vi "WSS.Generate.Digital.vi"(8 "Man Ctrl Bit 1":bool, 9 "Man Ctrl Bit 0":bool, 10 "Manual Control":bool, 11 "LF Wheel Speed Sensor Settings":T1={"ACTIVE EDGE"=TRUE, "ACTIVE TICKS"=0, "INACTIVE TICKS"=0, "Data"=0, "Sensor Type"=0}) -> (1 "Bit1":bool, 2 "Bit0":bool)   [LabVIEW 2015, in "Speciality FPGA IO.lvlib"]
doc: "This VI Simulates Wheel Speed Sensors for Unidirectional, Bidirectional - Bosch, and Bidirectional Conti. Sensor Type is:\n0 - Unidirectional\n1 - Bidirectional Bosch\n2 - Bidirectional Continental. The output of the VI is two digital bits that correspond to the following current levels when paired with an OW-902 module:\nBit 0 Bit 1 Output Current Level\n0 0 0\n0 1 Lo\n1 0 Mid\n1 1 Hi"
uses:
  Speciality FPGA IO.lvlib
  Types/PWM.Generate.Digital.Settings.ctl
  Types/WSS.Generate.Digital.Settings.ctl
panel:
  out "Data Played Out":bool[](array[boolean])
  out "Boolean array":bool[](array[boolean])
  # "M\nS\nB"
  # "L\nS\nB"
  # "P\na\nr\ni\nt\ny"
  # "Only 9 bits played out"
  # "M\nS\nB"
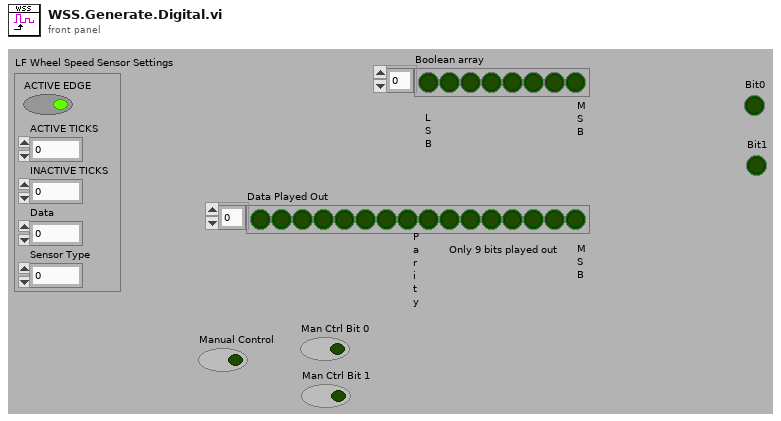
[diagram p1: front panel]
types:
  T1 = typedef "Speciality FPGA IO.lvlib/WSS.Generate.Digital.Settings.ctl" = cluster{"ACTIVE EDGE":bool, "ACTIVE TICKS":u32, "INACTIVE TICKS":u32, "Data":u8, "Sensor Type":u8}
  T2 = typedef "Speciality FPGA IO.lvlib/PWM.Generate.Digital.Settings.ctl" = cluster{"ACTIVE EDGE":bool, "ACTIVE TICKS":u32, "INACTIVE TICKS":u32}
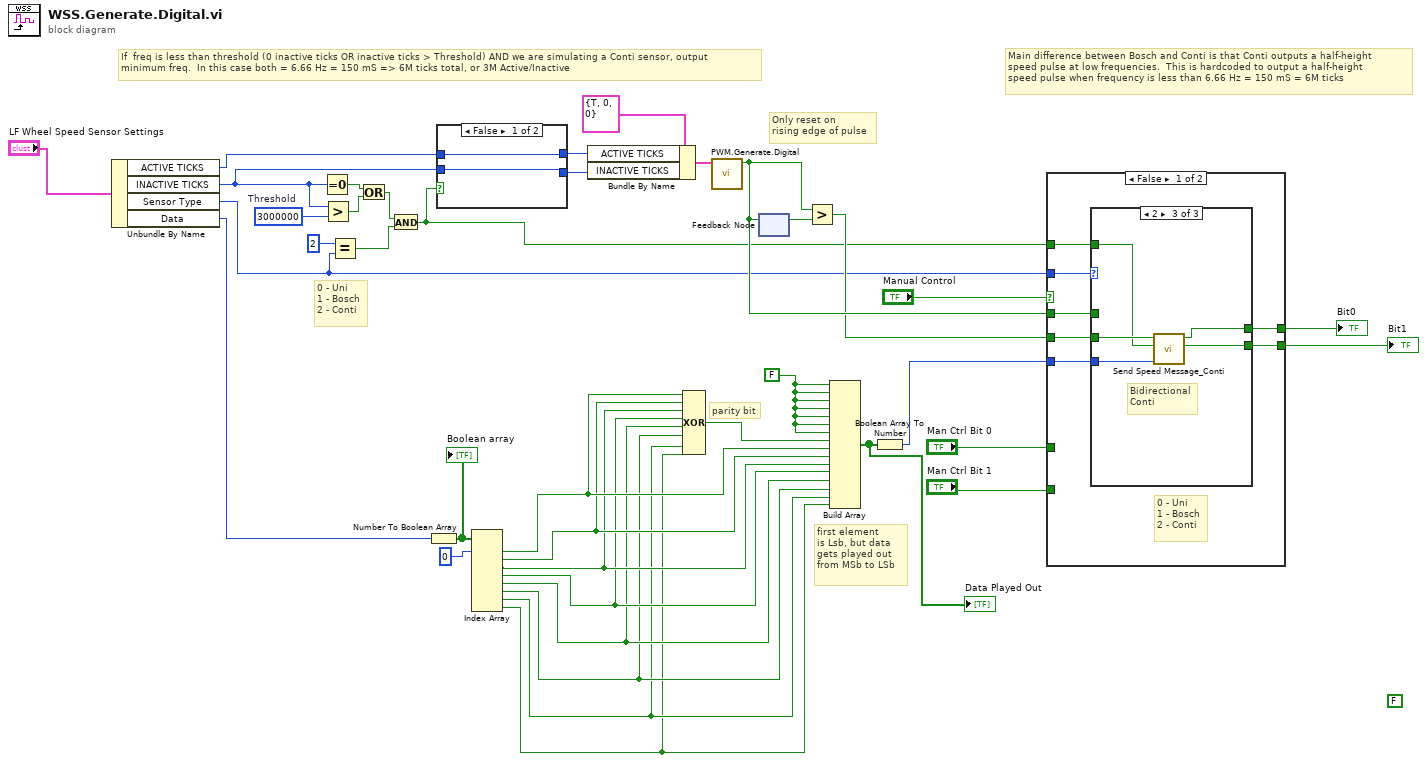
[diagram p0: block diagram]
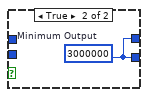
[diagram p2: hidden frame]
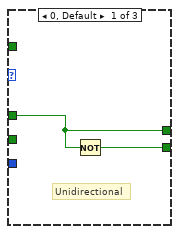
[diagram p3: hidden frame]
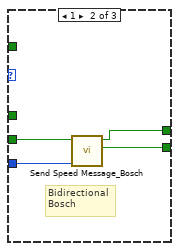
[diagram p4: hidden frame]
diagram:
  w19 = u32 3000000  # Threshold
  w36 = FALSE ("element")
  (unwired) FALSE
  # "first element\nis Lsb, but data \ngets played out \nfrom MSb to LSb"
  # "Only reset on\nrising edge of pulse"
  # "0 - Uni\n1 - Bosch\n2 - Conti"
  # "If  freq is less than threshold (0 inactive ticks OR inactive ticks > Threshold) AND we are simulating a Conti sensor, output \nminimum freq.  In this case both = 6.66 Hz = 150 mS => 6M ticks total, or 3M Active/Inactive"
  # "Main difference between Bosch and Conti is that Conti outputs a half-height\nspeed pulse at low frequencies.  This is hardcoded to output a half-height\nspeed pulse when frequency is less than 6.66 Hz = 150 mS = 6M ticks"
  # "parity bit"
  n1 = Unbundle By Name("LF Wheel Speed Sensor Settings") -> ("ACTIVE TICKS"=w6:u32, "INACTIVE TICKS"=w5:u32, "Sensor Type"=w8:u8, "Data"=w14:u8)
  n2 = Equal To 0?(x=w5) -> (x = 0?=w11:bool)
  n3 = Greater?(x=w5, y=w19) -> (0:w10:bool)
  n4 = Equal?(x=u8 2, y=w8) -> (x = y?=w20:bool)
  n5 = Or(x=w11, y=w10) -> (x .or. y?=w9:bool)
  n6 = And(x=w9, y=w20) -> (x .and. y?=w7:bool)
  n7 = Number To Boolean Array(number=w14) -> (Boolean array=w30:bool[])
  "Boolean array" <- w30
  n8 = case shown="False" w7 {
    tunnel: [w39 w41] -> w4
    tunnel: [w40 w41] -> w3
    tunnel: w6 -> [w40 _]
    tunnel: w5 -> [w39 _]
    frame False {
    }
    frame True {
      w41 = u32 3000000  # Minimum Output
    }
  }
  n9 = Index Array(array=w30, index #1=0 ("index")) -> (element #1=w28:bool, element #2=w27:bool, element #3=w26:bool, element #4=w25:bool, element #5=w24:bool, element #6=w23:bool, element #7=w22:bool, element #8=w21:bool)  [unwired: 7 in]
  n10 = Bundle By Name(cluster=T2 {"ACTIVE EDGE"=TRUE, "ACTIVE TICKS"=0, "INACTIVE TICKS"=0} ("Settings"), "ACTIVE TICKS"=w3, "INACTIVE TICKS"=w4) -> (w12:T2)
  n11 = Compound Arithmetic op=XOR(w28, w27, w26, w25, w24, w23, w22, w21) -> (w31:bool)
  n12 = call "PWM.Generate.Digital.vi"("Settings"=w12) -> ("Output"=w18:bool)  [unwired: 10 in]
  n13 = feedback #1() -> (w35:bool)  [unwired: 1 in]
  n14 = feedback-in #1(w18) -> ()
  n15 = Greater?(x=w18, y=w35) -> (0:w17:bool)
  n16 = Build Array(w36, w36, w36, w36, w36, w36, w36, w31, w28, w27, w26, w25, w24, w23, w22, w21) -> (w38:bool[])
  "Data Played Out" <- w38
  n17 = Boolean Array To Number(Boolean array=w38) -> (number=w37:u16)
  n18 = case shown="False" "Manual Control" {
    tunnel: [w46 w61] -> w2
    tunnel: [w45 w60] -> w1
    tunnel: w37 -> [w48 _]
    tunnel: w17 -> [w47 _]
    tunnel: "Man Ctrl Bit 0" -> [_ w61]
    tunnel: "Man Ctrl Bit 1" -> [_ w60]
    tunnel: w18 -> [w44 _]
    tunnel: w8 -> [w43 _]
    tunnel: w7 -> [w42 _]
    frame False {
      # "0 - Uni\n1 - Bosch\n2 - Conti"
      n19 = case shown="2" w43 {
        tunnel: w48 -> [_ w54 w59]
        tunnel: w47 -> [_ w53 w58]
        tunnel: [w49 w52 w57] -> w46
        tunnel: [w50 w51 w56] -> w45
        tunnel: w44 -> [w49 _ _]
        tunnel: w42 -> [_ _ w55]
        frame 0, Default {
          # "Unidirectional"
          n20 = Not(x=w49) -> (.not. x?=w50:bool)
        }
        frame 1 {
          # "Bidirectional\nBosch"
          n21 = call "Send Speed Message_Bosch.vi"("Data"=w54, "Reset"=w53) -> ("Bit 1 Out"=w51:bool, "Bit 0 Out"=w52:bool)  [unwired: 6 in]
        }
        frame 2 {
          # "Bidirectional\nConti"
          n22 = call "Send Speed Message_Conti.vi"("Data"=w59, "Standstill"=w55, "Reset"=w58) -> ("Bit 1 Out"=w56:bool, "Bit 0 Out"=w57:bool)  [unwired: 5 in]
        }
      }
    }
    frame True {
    }
  }
  "Bit0" <- w2
  "Bit1" <- w1
